vi "process waveplate string.vi"(8 "error in (no error)":errorcluster, 11 "Simulated_CCD_Camera in":refnum<class "Simulated_CCD_Camera.lvclass">) -> (0 "error out":errorcluster, 3 "Simulated_CCD_Camera out":refnum<class "Simulated_CCD_Camera.lvclass">)   [LabVIEW 2018, in "Simulated_CCD_Camera.lvclass"]
uses:
  Simulated_CCD_Camera.lvclass
  Simulated_CCD_Camera.lvclass/Simulated_CCD_Camera.ctl
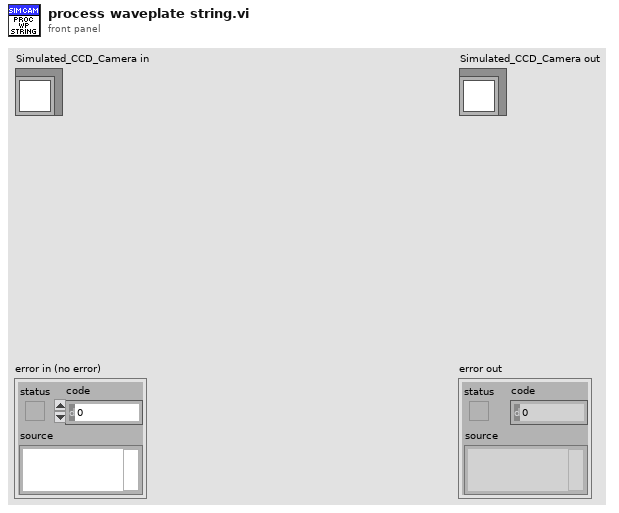
[diagram p1: front panel]
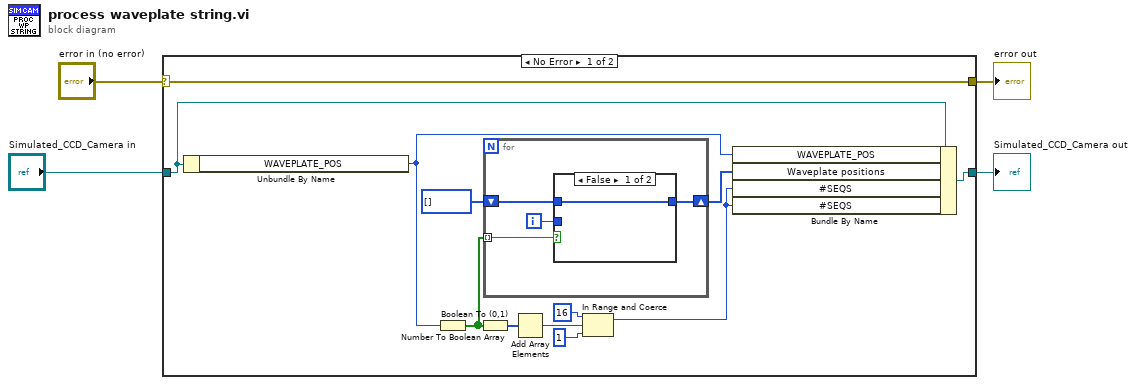
[diagram p0: block diagram]
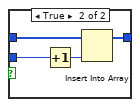
[diagram p2: hidden frame]
diagram:
  n1 = case shown="No Error" "error in (no error)" {
    selector: "error in (no error)" -> [w16 w27]
    tunnel: [w16 w27] -> w3
    tunnel: [w14 w26] -> w1
    tunnel: "Simulated_CCD_Camera in" -> [w15 w26]
    frame No Error {
      n2 = Unbundle By Name(w15) -> ("WAVEPLATE_POS"=w5:u16)
      n3 = Number To Boolean Array(number=w5) -> (Boolean array=w13:bool[])
      n4 = Boolean To (0,1)(Boolean=w13) -> (0, 1=w12:i16[])
      n5 = for {
        tunnel: w13 -> [w17] mode=indexing
        shift-right: [w18] -> w10
        shift-left: i32[] [] -> [w20]
        i -> [w19]
        n6 = case shown="False" w17 {
          tunnel: w20 -> [w21 w25]
          tunnel: w19 -> [_ w22]
          tunnel: [w21 w24] -> w18
          frame False {
          }
          frame True {
            n7 = Increment(x=w22) -> (x+1=w23:i32)
            n8 = Insert Into Array(array=w25, new element=w23) -> (w24:i32[])  [unwired: 1 in]
          }
        }
      }
      n9 = Add Array Elements(numeric array=w12) -> (sum=w9:i16)
      n10 = In Range and Coerce(upper limit=i16 16, x=w9, lower limit=i16 1) -> (coerced(x)=w6:i16)  [unwired: 1 out]
      n11 = Bundle By Name(cluster=w15, "WAVEPLATE_POS"=w5, "Waveplate positions"=w10, "#SEQS"=w6, "#SEQS"=w6) -> (w14:refnum<class "Simulated_CCD_Camera.lvclass">)
    }
    frame Error {
    }
  }
  "error out" <- w3
  "Simulated_CCD_Camera out" <- w1
